vi "Element Update Callback VI Type.vi"(7 "Owner":refnum<class>, 10 "Index":i32, 11 "Value":variant) -> ()   [LabVIEW 2020, in "Control Array.lvlib"]
uses:
  Control Array.lvlib
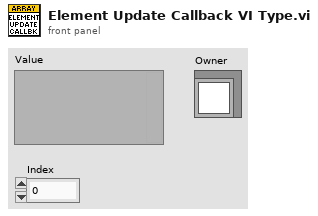
[diagram p1: front panel]
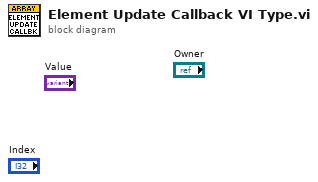
[diagram p0: block diagram]
diagram:
